vi "LWXPS_APIListAMATGet.vi"(0 "XPS Reference IN":refnum<k24>, 11 "LabVIEW error IN":errorcluster) -> (4 "XPS Reference OUT":refnum<k24>, 6 "Returned error code":i32, 8 "AMAT API method List":string, 10 "XPS Error String":string, 15 "LabVIEW error OUT":errorcluster)   [LabVIEW 2014]
uses:
  D:/XPSQ8_LabView_Library/Development/Source/Dll/Newport.XPS.CommandInterface.dll
  Dll/Newport.XPS.CommandInterface.dll
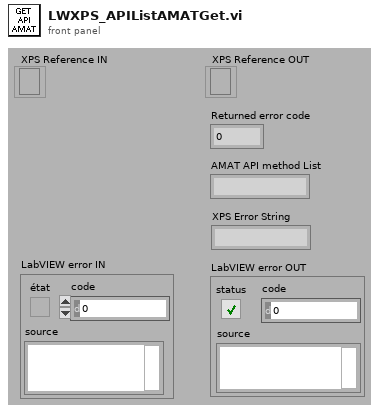
[diagram p1: front panel]
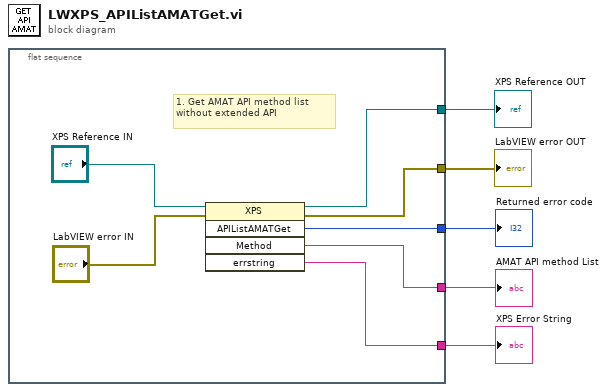
[diagram p0: block diagram]
diagram:
  n1 = flat-sequence {
    tunnel: [w10] -> w5
    tunnel: [w9] -> w4
    tunnel: [w8] -> w3
    tunnel: [w7] -> w2
    tunnel: [w6] -> w1
    frame #0 {
      # "1. Get AMAT API method list without extended API"
      n2 = invoke class="XPS" method="APIListAMATGet"(reference="XPS Reference IN", error in="LabVIEW error IN") -> (reference out=w10:refnum<k24>, error out=w9:errorcluster, "APIListAMATGet"=w6:i32, "Method"=w7:string, "errstring"=w8:string)  [unwired: 3 in]
    }
  }
  "XPS Reference OUT" <- w5
  "LabVIEW error OUT" <- w4
  "XPS Error String" <- w3
  "AMAT API method List" <- w2
  "Returned error code" <- w1
